vi "JAS_CameraSimCameraRead.vi"(7 "Operation":enum16{"Read", "Reopen", "Close"}(ring), 8 "error in":errorcluster, 10 "address":string="10.te.am.11", 11 "Image":T1) -> (0 "error out":errorcluster, 1 "Reconnect":bool, 2 "length":i32, 3 "Image Out":T1)   [LabVIEW 2025]
doc: "This VI is intended for testing, examples, and demos. It assumes the camera is directly accssible from the computer and not the robot. It retrieves an image from either a USB or IP Axis camera.\n\nThis software is licensed. Open the labview\\readme\\WPI Robotics Library Open Source License.txt file for more information."
uses:
  <vilib>/vision/Image Controls.llb/IMAQ Image.ctl
  <vilib>/picture/picture.llb/imagedata.ctl
  JAS_CameraImageSize.ctl
  JAS_CameraSettings Read MJPG.ctl
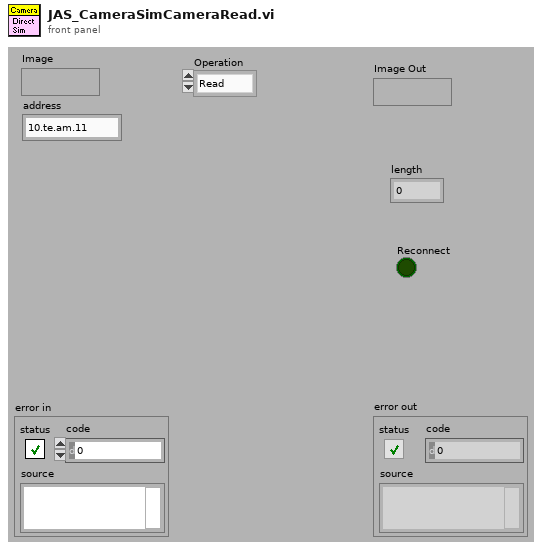
[diagram p1: front panel]
types:
  T1 = typedef "IMAQ Image.ctl" = refnum<image>
  T2 = typedef "JAS_CameraSettings Read MJPG.ctl" = cluster{"fps":i32, "compression":i32, "Image Size":T3, "Config Shown":bool}
  T3 = typedef "JAS_CameraImageSize.ctl" = enum16{"640x480", "640x360", "320x240", "320x180", "160x120", "160x90", "Custom"}
  T4 = typedef "imagedata.ctl" = cluster{"image type":i32, "image depth":i32, "image":u8[], "mask":u8[], "colors":u32[], "Rectangle":cluster{"left":i16, "top":i16, "right":i16, "bottom":i16}}
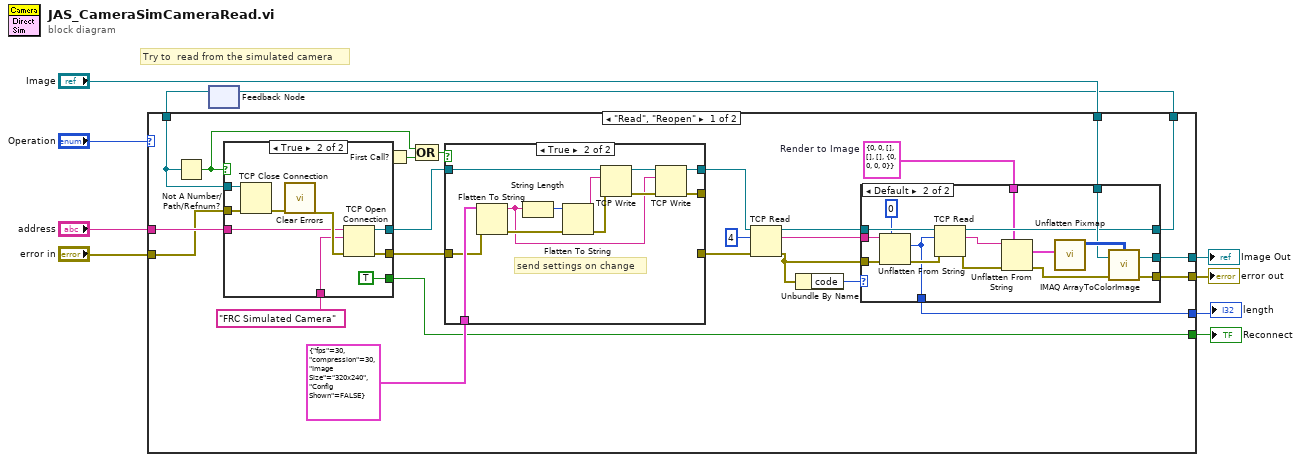
[diagram p0: block diagram]
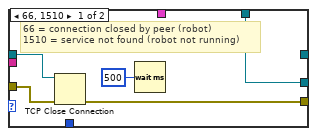
[diagram p3: hidden frame]
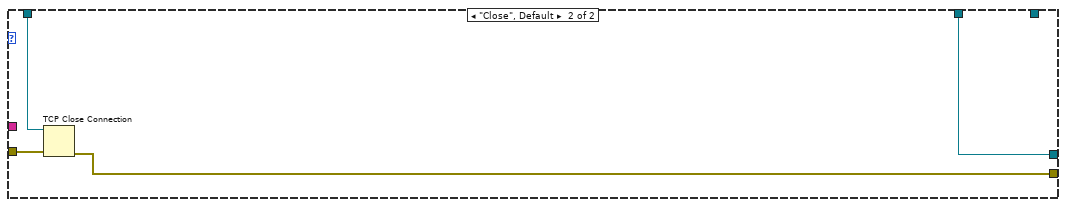
[diagram p5: hidden frame]
diagram:
  # "Try to  read from the simulated camera"
  n1 = feedback #1() -> (w3:refnum<k5>)  [unwired: 1 out]
  n2 = case shown="\"Read\", \"Reopen\"" "Operation" {
    tunnel: "address" -> [w34 _]
    tunnel: "error in" -> [w33 w84]
    tunnel: [w32 w82] -> w8
    tunnel: [w24 w83] -> w5
    tunnel: "Image" -> [w31 w82]
    tunnel: [w26 _] -> w2
    tunnel: [w25 _] -> w4
    tunnel: w3 -> [w14 w81]
    tunnel: [w11 _] -> w1
    frame "Read", "Reopen" {
      w13 = T4 {"image type"=0, "image depth"=0, "image"=[], "mask"=[], "colors"=[], "Rectangle"={"left"=0, "top"=0, "right"=0, "bottom"=0}}  # Render to Image
      n3 = Not A Number/Path/Refnum?(number/path/refnum=w14) -> (NaN/Path/Refnum?=w21:bool)
      n4 = case shown="True" w21 {
        tunnel: w14 -> [w71 w80]
        tunnel: w34 -> [_ w74]
        tunnel: [w71 w77] -> w20
        tunnel: w33 -> [w70 w76]
        tunnel: [w70 w75] -> w18
        tunnel: "FRC Simulated Camera" ("service name") -> [_ w73]
        tunnel: [_ TRUE] -> w11
        frame False {
        }
        frame True {
          n5 = TCP Close Connection(connection ID=w80, error in (no error)=w76) -> (error out=w79:errorcluster)  [unwired: 2 out]
          n6 = call <vilib>:"Clear Errors.vi"("error in (no error)"=w79) -> ("error out"=w78:errorcluster)  [unwired: 1 in, 5 out]
          n7 = TCP Open Connection(address=w74, remote port or service name=w73, error in (no error)=w78) -> (connection ID=w77:refnum<k5>, error out=w75:errorcluster)  [unwired: 2 in]
        }
      }
      n8 = First Call?() -> (First Call?: T/F=w23:bool)
      n9 = Compound Arithmetic op=OR(w21, w23) -> (w22:bool)
      n10 = case shown="True" w22 {
        tunnel: w20 -> [w36 w48]
        tunnel: T2 {"fps"=30, "compression"=30, "Image Size"=enum."320x240", "Config Shown"=FALSE} ("Camera Settings") -> [_ w46]
        tunnel: [w36 w39] -> w19
        tunnel: w18 -> [w35 w38]
        tunnel: [w35 _] -> w17
        tunnel: [_ w37] -> _
        frame False {
        }
        frame True {
          # "send settings on change"
          n11 = Flatten To String(anything=w46, error in (no error)=w38) -> (data string=w40:string, error out=w42:errorcluster)  [unwired: 2 in, 1 out]
          n12 = String Length(string=w40) -> (length=w47:i32)
          n13 = Flatten To String(anything=w47, error in (no error)=w42) -> (data string=w45:string, error out=w43:errorcluster)  [unwired: 2 in, 1 out]
          n14 = TCP Write(connection ID=w48, data in=w45, error in (no error)=w43) -> (connection ID out=w41:refnum<k5>, error out=w44:errorcluster)  [unwired: 1 in, 1 out]
          n15 = TCP Write(connection ID=w41, data in=w40, error in (no error)=w44) -> (connection ID out=w39:refnum<k5>, error out=w37:errorcluster)  [unwired: 1 in, 1 out]
        }
      }
      n16 = TCP Read(connection ID=w19, bytes to read=4, error in (no error)=w17) -> (connection ID out=w28:refnum<k5>, data out=w29:string, error out=w15:errorcluster)  [unwired: 1 in, 1 out]
      n17 = Unbundle By Name(w15) -> ("code"=w27:i32)
      n18 = case shown="Default" w27 {
        tunnel: [w53 w66] -> w32
        tunnel: [w49 w55] -> w24
        tunnel: w31 -> [w53 w65]
        tunnel: w29 -> [_ w64]
        tunnel: w28 -> [w51 w63]
        tunnel: w15 -> [w50 w61]
        tunnel: [_ w59] -> w26
        tunnel: [_ w56] -> w25
        tunnel: w13 -> [_ w54]
        frame 66, 1510 {
          # "66 = connection closed by peer (robot)\n1510 = service not found (robot not running)"
          n19 = TCP Close Connection(connection ID=w51, error in (no error)=w50) -> (error out=w49:errorcluster)  [unwired: 2 out]
          n20 = Wait (ms)(milliseconds to wait=u32 500) -> ()  [unwired: 1 out]
        }
        frame Default {
          n21 = Unflatten From String(type=0 ("bytes to read"), binary string=w64, error in (no error)=w61) -> (value=w59:i32, error out=w60:errorcluster)  [unwired: 2 in, 1 out]
          n22 = TCP Read(connection ID=w63, bytes to read=w59, error in (no error)=w60) -> (connection ID out=w56:refnum<k5>, data out=w67:string, error out=w58:errorcluster)  [unwired: 1 in, 1 out]
          n23 = Unflatten From String(type=w54, binary string=w67, error in (no error)=w58) -> (value=w68:T4, error out=w57:errorcluster)  [unwired: 2 in, 1 out]
          n24 = call <vilib>:"Unflatten Pixmap.vi"("image data"=w68) -> ("24-bit pixmap"=w69:u32[][])  [unwired: 4 in, 6 out]
          n25 = call "IMAQ ArrayToColorImage"("Image Pixels (U32)"=w69, "Image"=w65, "error in (no error)"=w57) -> ("Image Out"=w66:T1, "error out"=w55:errorcluster)  [unwired: 2 in]
        }
      }
    }
    frame "Close", Default {
      n26 = TCP Close Connection(connection ID=w81, error in (no error)=w84) -> (error out=w83:errorcluster)  [unwired: 2 out]
    }
  }
  "Image Out" <- w8
  "error out" <- w5
  "length" <- w2
  "Reconnect" <- w1
  n27 = feedback-in #1(w4) -> ()
